vi "Convert Single to U8.vi"(1 "Image Pixels (Float)":sgl[][](array[numeric])) -> (0 "Image Pixels (U8)":u8[][](array[numeric]))   [LabVIEW 2019, in "BigMAQ.lvclass"]
uses:
  BigMAQ.lvclass
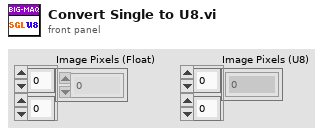
[diagram p1: front panel]
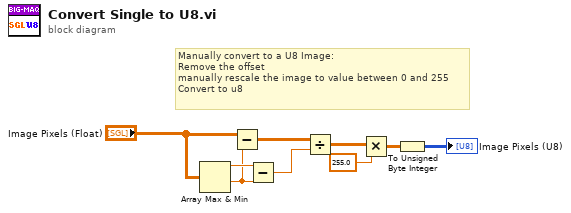
[diagram p0: block diagram]
diagram:
  # "Manually convert to a U8 Image:\nRemove the offset\nmanually rescale the image to value between 0 and 255\nConvert to u8"
  n1 = Array Max & Min(array="Image Pixels (Float)") -> (max value=w9:sgl, min value=w3:sgl)  [unwired: 2 out]
  n2 = Subtract(x="Image Pixels (Float)", y=w3) -> (x-y=w4:sgl[][])
  n3 = Subtract(x=w9, y=w3) -> (x-y=w8:sgl)
  n4 = Divide(x=w4, y=w8) -> (x/y=w5:sgl[][])
  n5 = Multiply(x=sgl 255.0 ("x-y"), y=w5) -> (x*y=w6:sgl[][])
  n6 = To Unsigned Byte Integer(number=w6) -> (unsigned 8bit integer=→"Image Pixels (U8)":u8[][])
